vi "DB Import Action - Create Chans.vi"(8 "error in (no error)":errorcluster, 10 "selected path":path, 11 "Node Ptr":u64) -> (0 "error out":errorcluster, 2 "selected path out":path caption="selected path", 3 "Node Ptr dup":u64)   [LabVIEW 2020, in "Ballard 1553 System Explorer.lvlib"]
uses:
  Ballard 1553 System Explorer.lvlib
  Shared/Controls and Global/Global.vi
  <vilib>/NI VeriStand/Custom Device API/NI VeriStand - Add Custom Device Section.vi
  Create Sysdef Tree from DB Channel Clusters_BC.vi
  Create Sysdef Tree from DB Channel Clusters_RTs.vi
  <vilib>/NI VeriStand/Custom Device API/Set Item Property (Boolean).vi
  <vilib>/NI VeriStand/Custom Device API/Custom Device API.lvlib
  Shared/Ballard 1553 Shared.lvlib
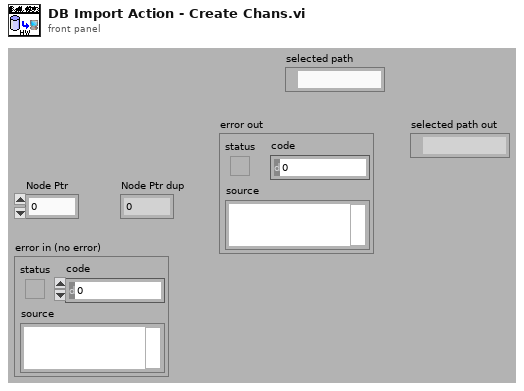
[diagram p1: front panel]
types:
  T1 = typedef "Ballard 1553 System Explorer.lvlib/Ballard_Channel.ctl" = cluster{"hardwareChannel":i32, "name":string, "BC":T2, "RTs":T10[], "ID":i32, "amplitudePercent":dbl, "broadcast":bool}
  T2 = typedef "Ballard 1553 System Explorer.lvlib/Ballard_BC.ctl" = cluster{"ID":i32, "name":string, "messageBuffers":cluster{"ID":i32, "name":string, "messageData":u16[]}[], "messages":T3[], "minorFrames":T7[], "majorFrames":T8[], "acyclicFrames":T9[]}
  T3 = typedef "Ballard 1553 System Explorer.lvlib/Ballard_message.ctl" = cluster{"ID":i32, "name":string, "messageBufferIDRef":i32, "messageType":T4, "CWD1":T5, "CWD2":T6}
  T4 = typedef "Ballard 1553 System Explorer.lvlib/Ballard_messageType.ctl" = enum16{"BC to RT", "RT to BC", "RT to RT", "MC (Rx)", "MC (Tx)"}
  T5 = typedef "Ballard 1553 System Explorer.lvlib/Ballard_CWD1.ctl" = cluster{"TA (RT)":i8, "SA":i8, "Mode Code":i8, "Words Count":i8}
  T6 = typedef "Ballard 1553 System Explorer.lvlib/Ballard_CWD2.ctl" = cluster{"TA (RT)":i8, "SA":i8, "Words (WC)":i8}
  T7 = typedef "Ballard 1553 System Explorer.lvlib/Ballard_minorFrame.ctl" = cluster{"ID":i32, "name":string, "frameTime":i32, "messageIDRefs":i32[]}
  T8 = typedef "Ballard 1553 System Explorer.lvlib/Ballard_majorFrame.ctl" = cluster{"ID":i32, "name":string, "loopCount":i32, "minorFrameIDRef":i32[]}
  T9 = typedef "Ballard 1553 System Explorer.lvlib/Ballard_acyclicFrame.ctl" = cluster{"ID":i32, "name":string, "messageIDRefs":i32[]}
  T10 = typedef "Ballard 1553 System Explorer.lvlib/Ballard_RT.ctl" = cluster{"ID":i32, "name":string, "rtAddress":i8, "responseTime":i32, "messageBuffers":cluster{"ID":i32, "name":string, "messageData":u16[]}[], "subAddresses":T11[], "rtMode":T13, "initialSwd":u16, "modeCodes":T14[]}
  T11 = typedef "Ballard 1553 System Explorer.lvlib/Ballard_RT subAddress.ctl" = cluster{"ID":i32, "name":string, "messageBufferIDRef":i32, "subAddress":i8, "direction":T12}
  T12 = typedef "Ballard 1553 System Explorer.lvlib/Ballard_RT direction.ctl" = enum16{"Tx", "Rx"}
  T13 = typedef "Ballard 1553 System Explorer.lvlib/Ballard_RT rtMode.ctl" = enum16{"Simulate", "Monitor", "Disable"}
  T14 = typedef "Ballard 1553 System Explorer.lvlib/Ballard_RT modeCode.ctl" = cluster{"ID":i32, "name":string, "messageBufferIDRef":i32, "modeCodeNumber":i8, "direction":T12}
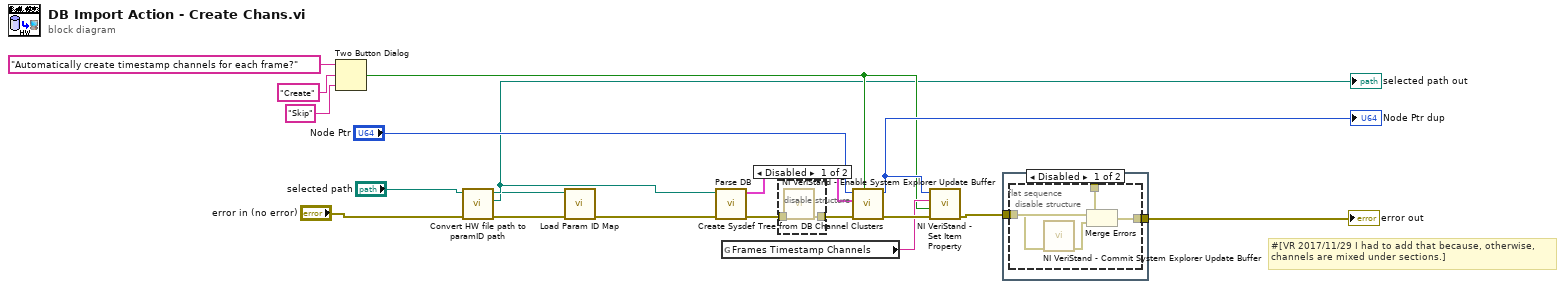
[diagram p0: block diagram]
diagram:
  # "#[VR 2017/11/29 I had to add that because, otherwise,\nchannels are mixed under sections.]"
  n1 = Two Button Dialog(message="Automatically create timestamp channels for each frame?", 1:"Skip" ("F button name (\"Cancel\")"), 2:"Create" ("T button name (\"OK\")")) -> (T button?=w8:bool)
  n2 = call "Convert HW file path to paramID path.vi"("error in (no error)"="error in (no error)", "Hw File In"="selected path") -> ("error out"=w2:errorcluster, "Param Id File out"=w3:path, "Hw File Out"=w4:path)  [unwired: 7 in]
  "selected path out" <- w4
  n3 = call "Load Param ID Map.vi"("error in (no error)"=w2, "Param Id File in"=w3) -> ("error out"=w1:errorcluster)  [unwired: 7 in, 2 out]
  n4 = call "Parse DB.vi"("error in (no error)"=w1, "Path in"=w4) -> ("error out"=w13:errorcluster, "channels"=w18:T1[])  [unwired: 8 in]
  n5 = global read "Global.vi" "Frames Timestamp Channels"() -> (w9:string)
  n6 = disable-structure shown="Disabled" {
    disable-tunnel: [w21 w22] -> w17
    disable-tunnel: w13 -> [w20 w22]
    frame Disabled {
      n7 = call <vilib>:"NI VeriStand - Enable System Explorer Update Buffer.vi"("error in (no error)"=w20) -> ("error out"=w21:errorcluster)  [unwired: 10 in]
    }
    frame Enabled {
    }
  }
  n8 = call "Create Sysdef Tree from DB Channel Clusters.vi"("Autocreate Rx timestamp chans?"=w8, "error in"=w17, "channels"=w18, "Device Ptr"="Node Ptr") -> ("error out"=w11:errorcluster, "Device Ptr dup"=w12:u64)  [unwired: 6 in]
  "Node Ptr dup" <- w12
  n9 = call-poly <vilib>:"NI VeriStand - Set Item Property.vi"("error in (no error)"=w11, "Value"=w8, "Property Name"=w9, "Item Ref in"=w12) -> ("error out"=w10:errorcluster)  [unwired: 5 in, 2 out]
  n10 = flat-sequence {
    tunnel: w10 -> [w23]
    tunnel: [w24] -> w7
    frame #0 {
      n11 = disable-structure shown="Disabled" {
        disable-tunnel: w23 -> [w28 _]
        disable-tunnel: [w26 w29] -> w24
        disable-tunnel: w23 -> [w25 w29]
        frame Disabled {
          n12 = call <vilib>:"NI VeriStand - Commit System Explorer Update Buffer.vi"("error in (no error)"=w25) -> ("error out"=w27:errorcluster)  [unwired: 10 in]
          n13 = Merge Errors(w28, w27) -> (w26:errorcluster)
        }
        frame Enabled {
        }
      }
    }
  }
  "error out" <- w7
